vi "DAQ Multi IO Init.vi"(8 "error in":errorcluster) -> (0 "error out":errorcluster, 3 "DAQ Ref Cluster":T1)   [LabVIEW 2021]
uses:
  controls/DAQ Refnums.ctl
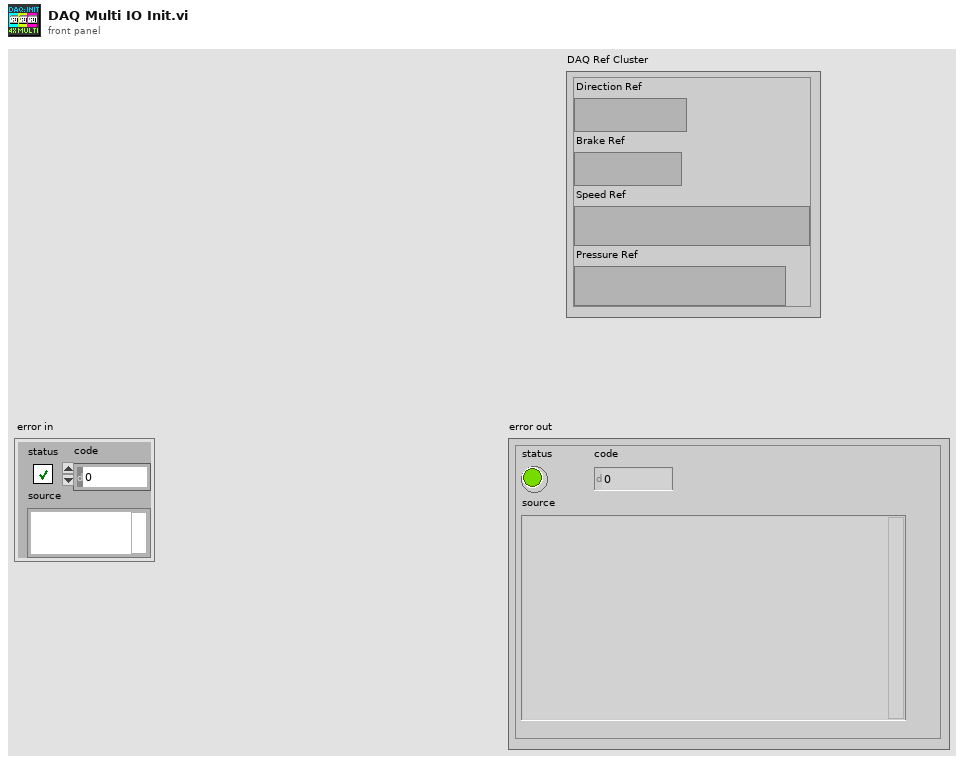
[diagram p1: front panel]
types:
  T1 = typedef "DAQ Refnums.ctl" = cluster{"Direction Ref":refnum<k21>, "Brake Ref":refnum<k21>, "Speed Ref":refnum<k21>, "Pressure Ref":refnum<k21>}
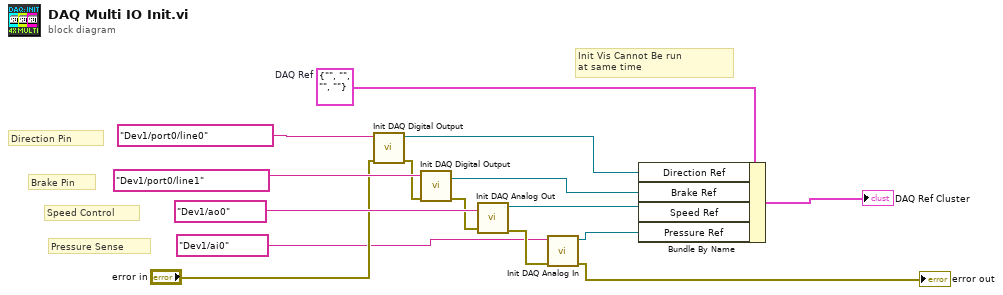
[diagram p0: block diagram]
diagram:
  w15 = T1 {"Direction Ref"="", "Brake Ref"="", "Speed Ref"="", "Pressure Ref"=""}  # DAQ Ref
  # "Pressure Sense"
  # "Init Vis Cannot Be run\nat same time"
  # "Speed Control"
  # "Direction Pin"
  # "Brake Pin"
  n1 = call "Init DAQ Digital Output.vi"("error in"="error in", "lines"=tag "Dev1/port0/line0") -> ("error out"=w10:errorcluster, "Refnum out"=w12:refnum<k21>)  [unwired: 8 in]
  n2 = call "Init DAQ Digital Output.vi"("error in"=w10, "lines"=tag "Dev1/port0/line1") -> ("error out"=w7:errorcluster, "Refnum out"=w13:refnum<k21>)  [unwired: 8 in]
  n3 = call "Init DAQ Analog Out.vi"("error in"=w7, "physical channels"=tag "Dev1/ao0") -> ("error out"=w4:errorcluster, "Refnum out"=w6:refnum<k21>)  [unwired: 8 in]
  n4 = call "Init DAQ Analog In.vi"("error in"=w4, "physical channels"=tag "Dev1/ai0") -> ("error out"=→"error out":errorcluster, "Refnum out"=w3:refnum<k21>)  [unwired: 8 in]
  n5 = Bundle By Name(cluster=w15, "Direction Ref"=w12, "Brake Ref"=w13, "Speed Ref"=w6, "Pressure Ref"=w3) -> (→"DAQ Ref Cluster":T1)
